vi "ClusterwitharrayI32.vi"(1 "Cluster In":cluster{"Array In":i32[], "Numeric Input":i32}, 2 "Base":i32) -> (0 "Cluster Out":cluster{"Array Out":i32[], "Numeric Output":i32})   [LabVIEW 2013]
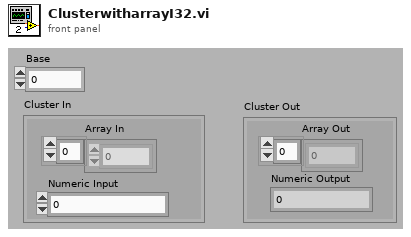
[diagram p1: front panel]
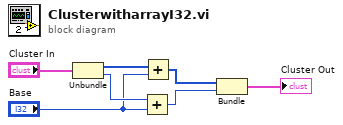
[diagram p0: block diagram]
diagram:
  n1 = Unbundle("Cluster In") -> ("Array In"=w7:i32[], "Numeric Input"=w6:i32)
  n2 = Add(x=w6, y="Base") -> (x+y=w4:i32)
  n3 = Add(x=w7, y="Base") -> (x+y=w5:i32[])
  n4 = Bundle(w5, w4) -> (→"Cluster Out":cluster{i32[], i32})  [unwired: 1 out]
